vi "CIMAQ_ResolveOptDst.vi"(9 "Dst(optional)":T1, 10 "Src":T1) -> (2 "Dst":T1, 3 "Src":T1)   [LabVIEW 2017]
uses:
  <vilib>/vision/Image Controls.llb/IMAQ Image.ctl
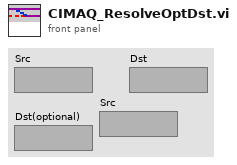
[diagram p1: front panel]
types:
  T1 = typedef "IMAQ Image.ctl" = refnum<image>
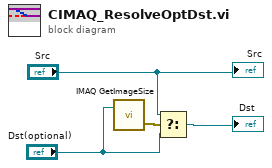
[diagram p0: block diagram]
diagram:
  n1 = call "IMAQ GetImageSize"("Image"="Dst(optional)") -> ("error out"=w2:errorcluster)  [unwired: 3 in, 2 out]
  n2 = Select(t="Src", s=w2, f="Dst(optional)") -> (s? t:f=→"Dst":T1)
  "Src" <- "Src"
